vi "Main.vi"(11 "Module Admin":refnum<class "Delacor_lib_QMH_Module Admin.lvclass">) -> ()   [LabVIEW 2021, in "HMI.lvlib"]
doc: "This template is based off of the Queued Message Handler design pattern and the Queued Message Handler project template that ships with LabVIEW.\n\nThe main difference is that the queue is private to this module and communication between modules is performed via Broadcast and Request events.\n\nRequest events are wrapped in public API methods and are handled in the Event Handling Loop (EHL) of this VI. Any module can register for Broadcast events sent by this module. The EHL generates messages based on user interface actions.\n\nThe Message Handling Loop (MHL) processes messages generated by the EHL, or by other messages. The messages are string values, so new messages can be added easily to the Message Cases case structure in the MHL. Each message cluster can also provide an optional value for Message Data, which is a variant that can be converted to whatever message-specific data is required.\n_____\nBased on DQMH Dev Tools: Project Template 7.1.2.1547."
uses:
  HMI.lvlib
  <vilib>/Delacor/Delacor QMH/Libraries/Module Admin_class/Delacor_lib_QMH_Module Admin.lvclass
  Module Data--cluster.ctl
  Get Measurement from UDP HL--cluster.ctl
  Stop Argument--cluster.ctl
  <vilib>/Delacor/Delacor QMH/Libraries/Message Queue_class/Delacor_lib_QMH_Message Queue.lvclass/Delacor_lib_QMH_Message Queue.ctl
  <vilib>/Delacor/Delacor QMH/Libraries/Module Admin_class/Delacor_lib_QMH_Module Admin.lvclass/Delacor_lib_QMH_Module Admin.ctl
  Open UDP Connection Argument--cluster.ctl
  <vilib>/Utility/miscctls.llb/LVPointTypeDef.ctl
  <vilib>/Delacor/Delacor QMH/Libraries/Message Queue_class/Delacor_lib_QMH_Enqueue Message (Single).vi
  <vilib>/Delacor/Delacor QMH/Libraries/Module Admin_class/Delacor_lib_QMH_Get External Launch.vi
  <vilib>/Delacor/Delacor QMH/Libraries/Message Queue_class/Delacor_lib_QMH_Message Queue.lvclass
panel:
  out "CPU 2 (%)":u8(slide) scale=0.0..100.0
  out "CPU 1 (%)":u8(slide) scale=0.0..100.0
  out "Memory ROM Available (%)":u8(slide) scale=0.0..100.0
  out "Memory RAM Available (%)":u8(slide) scale=0.0..100.0
  out "Record Time":dbl format="%<%H:%M:%S%3u>t"
  in  "Record TDMS File":bool
  out "Analog Input":dbl[](array[numeric])
  out "Digital Input":bool[](array[boolean])
  out "error out":errorcluster
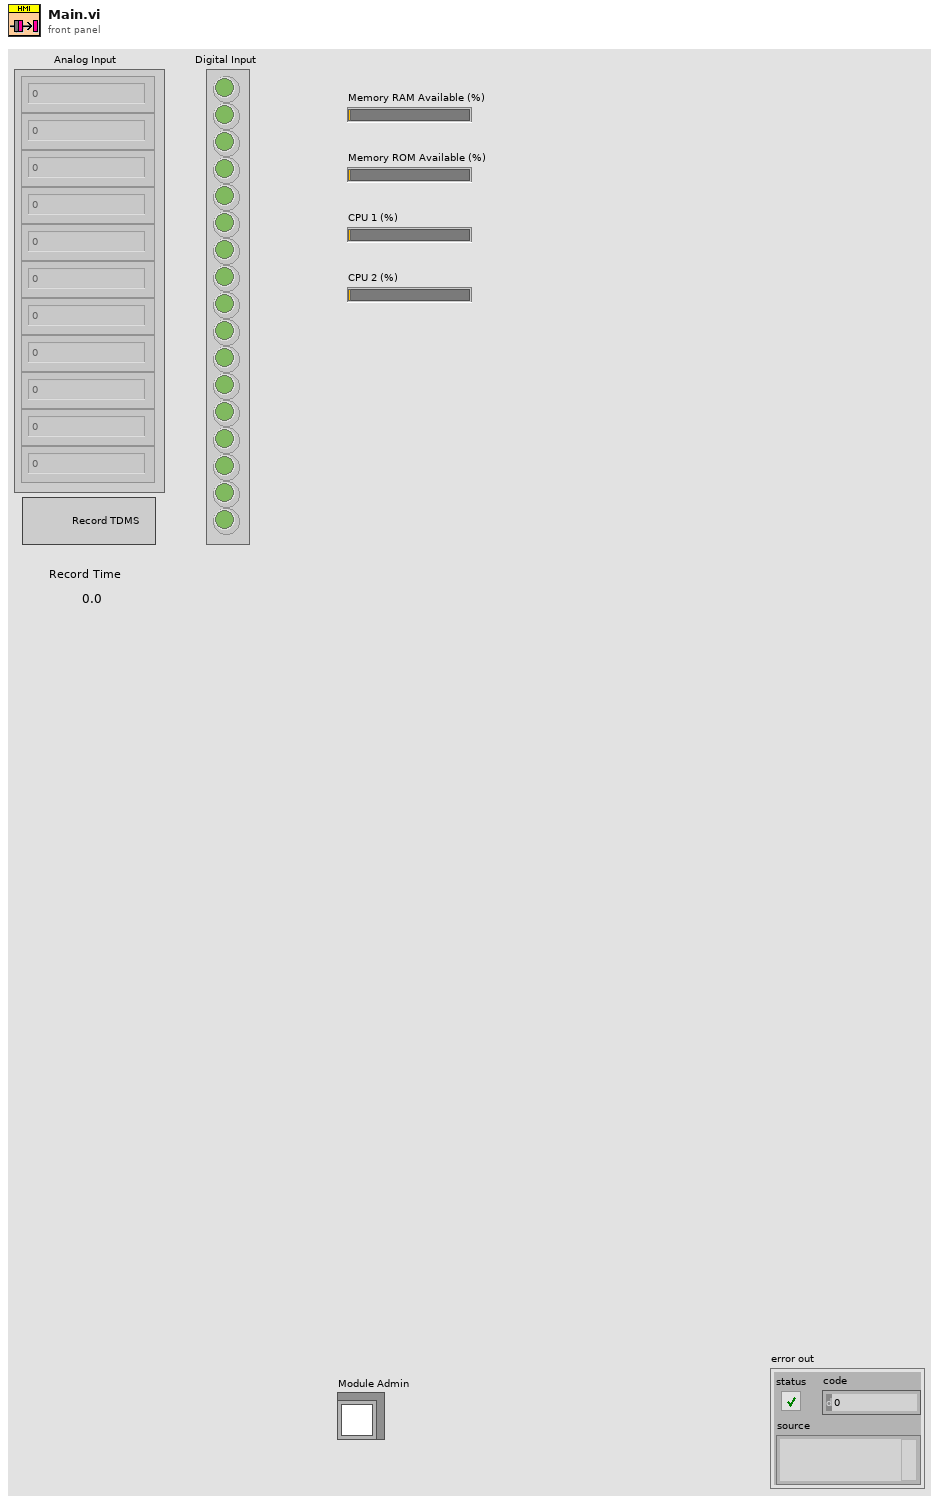
[diagram p1: front panel]
types:
  T1 = typedef "HMI.lvlib/Request Events--cluster.ctl" = cluster{"Stop Module":refnum<user-event>, "Show Panel":refnum<user-event>, "Hide Panel":refnum<user-event>, "Get Module Execution Status":refnum<user-event>, "Show Diagram":refnum<user-event>, "Private.Open UDP Connection":refnum<user-event>, "Private.Get UDP Info":refnum<user-event>, "Private.Recording":refnum<user-event>}
  T2 = typedef "HMI.lvlib/Get Measurement from UDP HL--cluster.ctl" = cluster{"IP RT":string, "Port RT":u16, "Port Host":u16, "connection ID":refnum<k16>, "Recording?":bool, "Timestamp":timestamp}
  T3 = typedef "HMI.lvlib/Module Data--cluster.ctl" = cluster{"Status":string, "IP RT":string, "Port RT":u16, "Port Host":u16, "connection ID":refnum<k16>}
  T4 = enum32{"invalid lock state", "Not Locked", "Locked (No Password)", "Password-protected"}
  T5 = typedef "HMI.lvlib/Stop Argument--cluster.ctl" = cluster{"Origin":string, "Exit via Stop Module Req?":bool, "Wait for Module to stop?":bool}
  T6 = typedef "HMI.lvlib/Open UDP Connection Argument--cluster.ctl" = cluster{"Boolean":bool}
  T7 = typedef "LVPointTypeDef.ctl" = cluster{"Horizontal":i16, "Vertical":i16}
  T8 = enum32{"Invalid", "Standard", "Closed", "Hidden", "Minimized", "Maximized"}
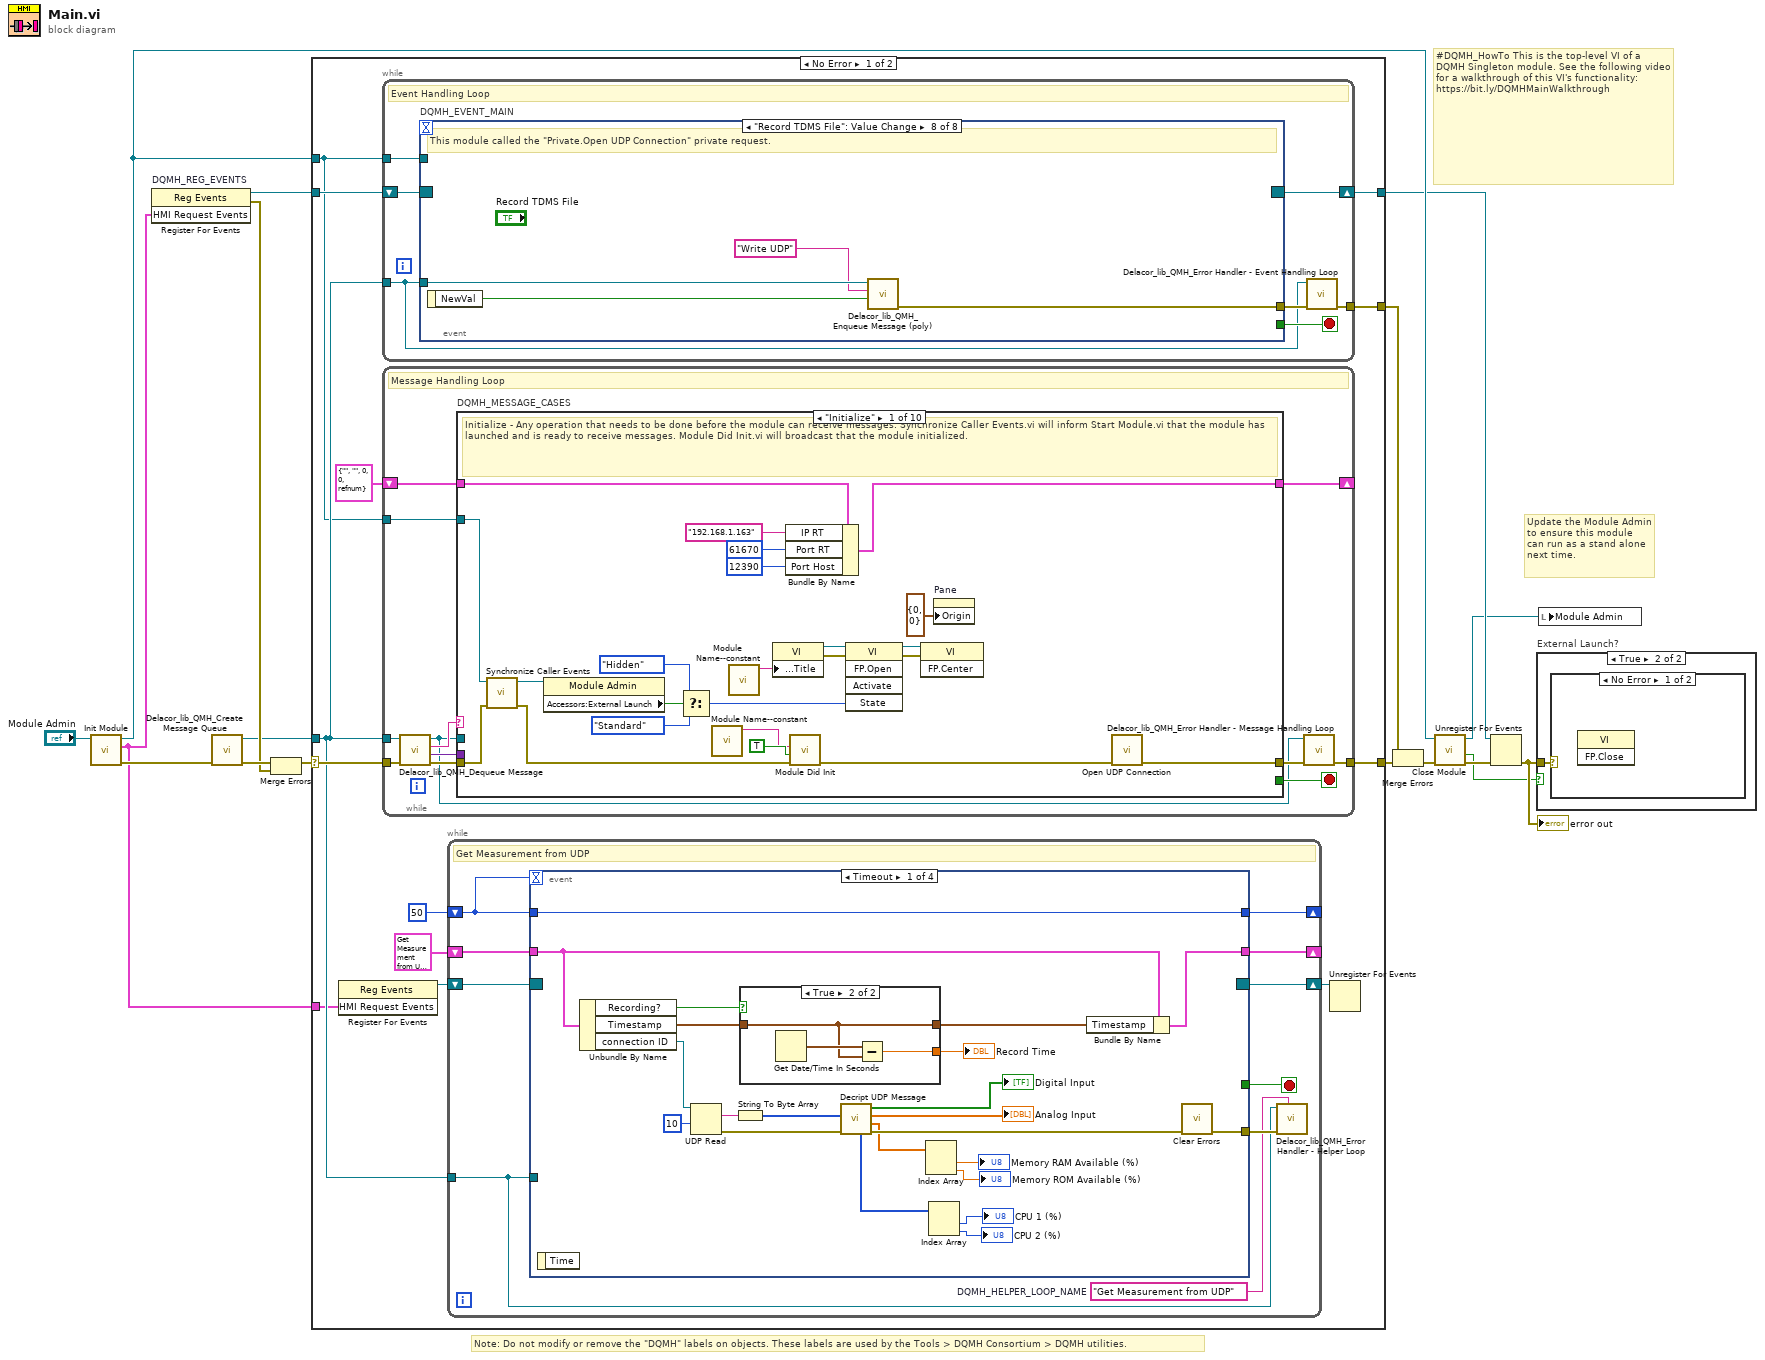
[diagram p0: block diagram]
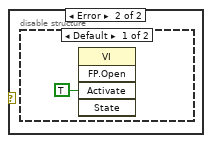
[diagram p3: hidden frame]
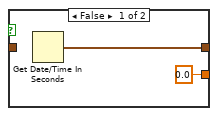
[diagram p5: hidden frame]
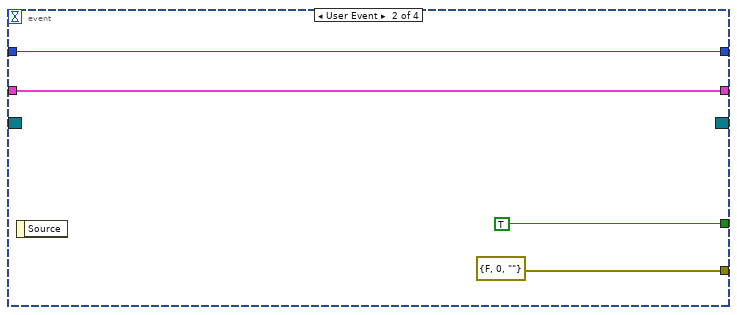
[diagram p6: hidden frame]
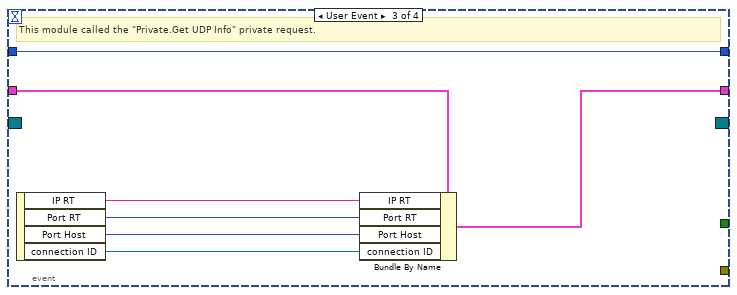
[diagram p7: hidden frame]
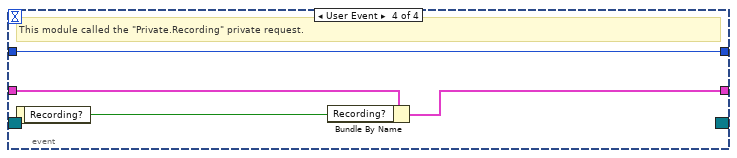
[diagram p8: hidden frame]
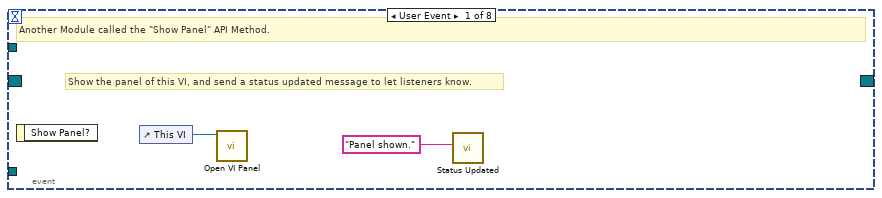
[diagram p9: hidden frame]
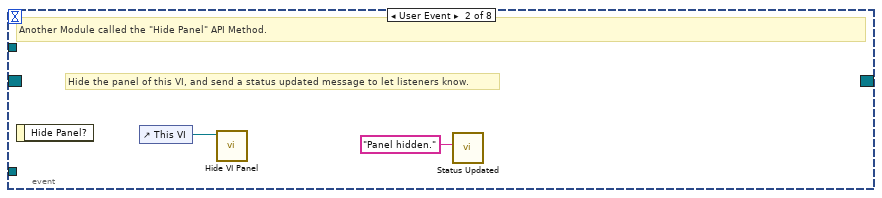
[diagram p10: hidden frame]
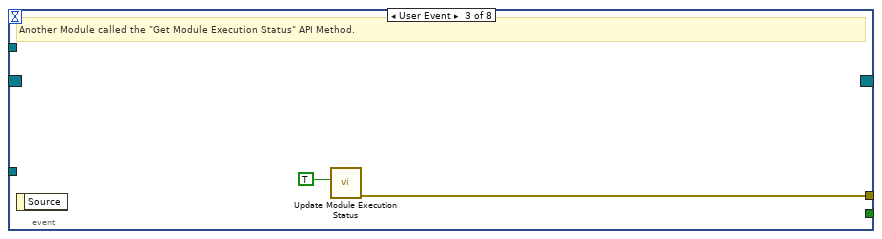
[diagram p11: hidden frame]
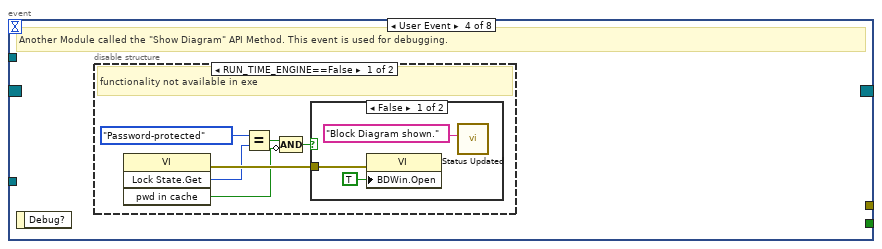
[diagram p12: hidden frame]
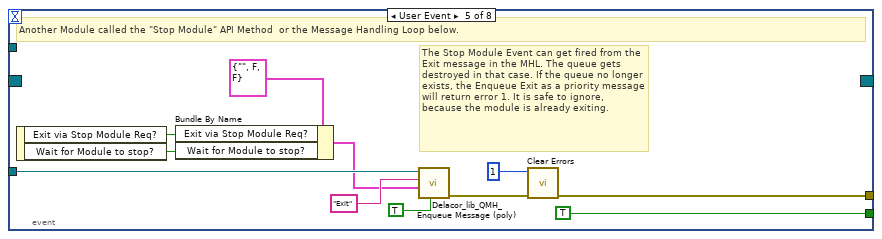
[diagram p15: hidden frame]
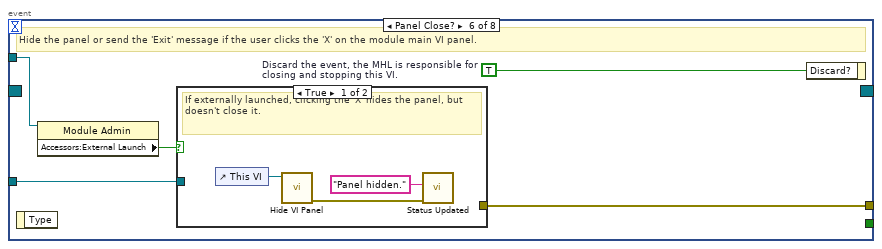
[diagram p16: hidden frame]
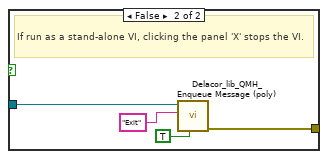
[diagram p17: hidden frame]
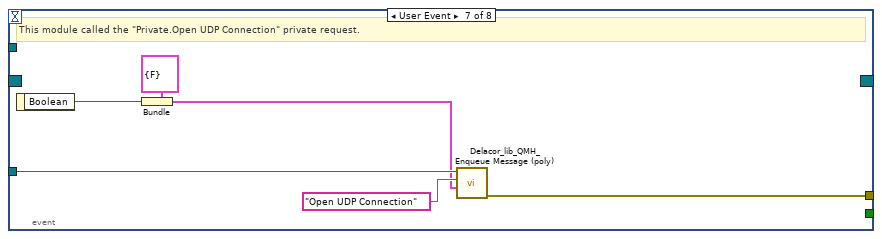
[diagram p18: hidden frame]
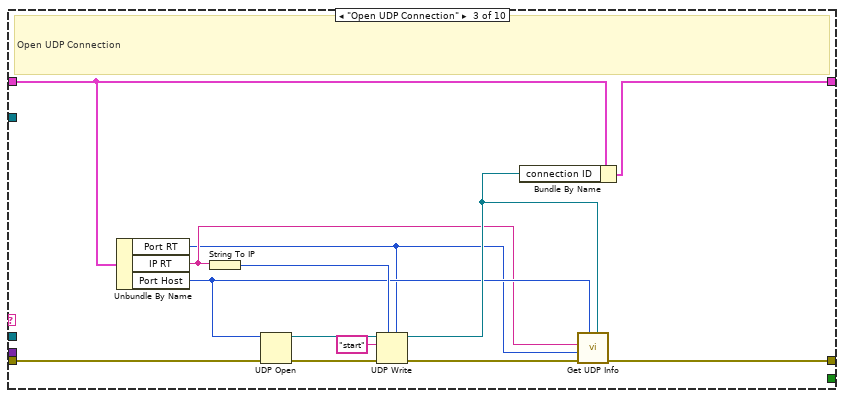
[diagram p20: hidden frame]
diagram:
  # "#DQMH_HowTo This is the top-level VI of a DQMH Singleton module. See the following video for a walkthrough of this VI's functionality: https://bit.ly/DQMHMainWalkthrough"
  # "Note: Do not modify or remove the \"DQMH\" labels on objects. These labels are used by the Tools > DQMH Consortium > DQMH utilities."
  # "Update the Module Admin to ensure this module can run as a stand alone next time."
  n1 = call "Init Module.vi"("Singleton Module Admin in"="Module Admin") -> ("error out"=w16:errorcluster, "HMI Request Events"=w1:T1, "Singleton Module Admin out"=w8:refnum<class "Delacor_lib_QMH_Module Admin.lvclass">)  [unwired: 8 in]
  n2 = register-events "DQMH_REG_EVENTS"(w1) -> (reference out=w6:refnum<event-registration>, error out=w9:errorcluster)  [unwired: 2 in]
  n3 = call <vilib>:"Delacor_lib_QMH_Create Message Queue.vi"("error in"=w16) -> ("error out"=w11:errorcluster, "Message Queue"=w5:refnum<class "Delacor_lib_QMH_Message Queue.lvclass">)  [unwired: 9 in]
  n4 = Merge Errors(w11, w9) -> (w10:errorcluster)
  n5 = case shown="No Error" w10 {
    selector: w10 -> [w28 w266]
    tunnel: [w30 w265] -> w17
    tunnel: [w27 w264] -> w7
    tunnel: w6 -> [w25 w264]
    tunnel: w5 -> [w24 w259]
    tunnel: [w29 _] -> w14
    tunnel: w8 -> [w23 w260]
    tunnel: w1 -> [w22 _]
    frame No Error {
      n6 = register-events ("DQMH_HELPER_REGFOREVENTS")(w22) -> (reference out=w20:refnum<event-registration>)  [unwired: 2 in, 1 out]
      n7 = while {
        tunnel: w24 -> [w83]
        shift-right: [w86] -> w27
        shift-left: w25 -> [w87]
        tunnel: [w88] -> w29
        tunnel: w23 -> [w84]
        stop <- w85 stop-if-true
        # "Event Handling Loop"
        n8 = event "DQMH_EVENT_MAIN" shown="[7] \"Record TDMS File\": Value Change" {
          selector: w87 -> [_ _ _ _ _ _ _ _]
          dyn-events: [_ _ _ _ _ _ _ _] -> w86
          timeout: _ -> [_ _ _ _ _ _ _ _]
          tunnel: [_ _ _ _ TRUE ("Discard?") _ _ _] -> w85
          tunnel: w83 -> [_ _ _ _ w111 w118 w133 w137]
          tunnel: [_ _ w95 _ w114 w120 w128 w135] -> w89
          tunnel: w84 -> [_ _ _ _ _ w117 _ _]
          event User Event {
            # "Show the panel of this VI, and send a status updated message to let listeners know."
            # "Another Module called the \"Show Panel\" API Method."
            n9 = event-data() -> ()  [unwired: 1 in, 1 out]
            n10 = control-ref of="This VI"() -> (w91:refnum<vi>)
            n11 = call "Open VI Panel.vi"("VI"=w91) -> ()  [unwired: 10 in, 1 out]
            n12 = call "Status Updated.vi"("Status"="Panel shown." ("format string")) -> ()  [unwired: 10 in, 1 out]
          }
          event User Event {
            # "Hide the panel of this VI, and send a status updated message to let listeners know."
            # "Another Module called the \"Hide Panel\" API Method."
            n13 = event-data() -> ()  [unwired: 1 in, 1 out]
            n14 = control-ref of="This VI"() -> (w93:refnum<vi>)
            n15 = call "Hide VI Panel.vi"("VI"=w93) -> ()  [unwired: 10 in, 1 out]
            n16 = call "Status Updated.vi"("Status"="Panel hidden." ("format string")) -> ()  [unwired: 10 in, 1 out]
          }
          event User Event {
            # "Another Module called the \"Get Module Execution Status\" API Method."
            n17 = event-data() -> ()  [unwired: 1 in, 1 out]
            n18 = call "Update Module Execution Status.vi"("Running?"=TRUE) -> ("error out"=w95:errorcluster)  [unwired: 10 in]
          }
          event User Event {
            # "Another Module called the \"Show Diagram\" API Method. This event is used for debugging."
            n19 = event-data() -> ()  [unwired: 1 in, 1 out]
            n20 = disable-structure shown="RUN_TIME_ENGINE==False" {
              frame condition #0 (active) {
                # "functionality not available in exe"
                n21 = invoke on="Invoke Node" class="VI" method="Lock State.Get"() -> (error out=w101:errorcluster, "Get Lock State"=w100:T4, "pwd in cache"=w97:bool)  [unwired: 4 in, 1 out]
                n22 = Equal?(x=T4."Password-protected", y=w100) -> (x = y?=w98:bool)
                n23 = Compound Arithmetic op=AND(w98, invert w97) -> (w96:bool)
                n24 = case shown="False" w96 {
                  tunnel: w101 -> [w104 _]
                  frame False {
                    n25 = property on="Property Node" class="VI"(error in=w104, "BDWin.Open"=TRUE ("Block Diagram Window:Open")) -> ()  [unwired: 1 in, 2 out]
                    n26 = call "Status Updated.vi"("Status"="Block Diagram shown." ("format string")) -> ()  [unwired: 10 in, 1 out]
                  }
                  frame True {
                    # "Password-protected VI, and the password is not in the cache. Do not show the diagram."
                  }
                }
              }
              frame condition #1 {
              }
            }
          }
          event User Event {
            # "The Stop Module Event can get fired from the Exit message in the MHL. The queue gets destroyed in that case. If the queue no longer exists, the Enqueue Exit as a priority message will return error 1. It is safe to ignore, because the module is already exiting."
            # "Another Module called the \"Stop Module\" API Method  or the Message Handling Loop below."
            n27 = event-data() -> ("Exit via Stop Module Req?"=w107:bool, "Wait for Module to stop?"=w106:bool)  [unwired: 1 in]
            n28 = Bundle By Name(cluster=T5 {"Origin"="", "Exit via Stop Module Req?"=FALSE, "Wait for Module to stop?"=FALSE} ("Stop Argument"), "Exit via Stop Module Req?"=w107, "Wait for Module to stop?"=w106) -> (w105:T5)
            n29 = call-poly <vilib>:"Delacor_lib_QMH_Enqueue Message (poly).vi"("Priority Message? (F)"=TRUE, "Message Data"=w105, "Message"="Exit", "Message Queue in"=w111) -> ("error out"=w115:errorcluster)  [unwired: 6 in, 1 out]
            n30 = call <vilib>:"Clear Errors.vi"("error in (no error)"=w115, "specific error code to clear (0: all)"=1) -> ("error out"=w114:errorcluster)  [unwired: 4 in, 1 out]
          }
          event Panel Close? {
            w119 = TRUE  # Discard the event, the MHL is responsible for closing and stopping this VI.
            # "Hide the panel or send the 'Exit' message if the user clicks the 'X' on the module main VI panel."
            n31 = event-data() -> ()  [unwired: 1 in, 1 out]
            n32 = property on="Property Node" class="Module Admin"(reference=w117) -> ("Accessors:External Launch"=w116:bool)  [unwired: 1 in, 2 out]
            n33 = case shown="True" w116 {
              tunnel: w118 -> [_ w126]
              tunnel: [_ w127] -> w120
              frame True {
                # "If externally launched, clicking the 'X' hides the panel, but doesn't close it."
                n34 = control-ref of="This VI"() -> (w123:refnum<vi>)
                n35 = call "Hide VI Panel.vi"("VI"=w123) -> ("error out"=w121:errorcluster)  [unwired: 10 in]
                n36 = call "Status Updated.vi"("error in"=w121, "Status"="Panel hidden." ("format string")) -> ()  [unwired: 9 in, 1 out]
              }
              frame False {
                # "If run as a stand-alone VI, clicking the panel 'X' stops the VI."
                n37 = call-poly <vilib>:"Delacor_lib_QMH_Enqueue Message (poly).vi"("Priority Message? (F)"=TRUE, "Message"="Exit", "Message Queue in"=w126) -> ("error out"=w127:errorcluster)  [unwired: 7 in, 1 out]
              }
            }
            n38 = event-data ("Event Filter Node")("Discard?"=w119) -> ()  [unwired: 1 in, 1 out]
          }
          event User Event {
            # "This module called the \"Private.Open UDP Connection\" private request."
            n39 = event-data() -> ("Boolean"=w129:bool)  [unwired: 1 in]
            n40 = Bundle(cluster=T6 {"Boolean"=FALSE} ("Open UDP Connection Argument"), "Boolean"=w129) -> (w130:T6)
            n41 = call-poly <vilib>:"Delacor_lib_QMH_Enqueue Message (poly).vi"("Message Data"=w130, "Message"="Open UDP Connection", "Message Queue in"=w133) -> ("error out"=w128:errorcluster)  [unwired: 7 in, 1 out]
          }
          event "Record TDMS File": Value Change {
            # "This module called the \"Private.Open UDP Connection\" private request."
            n42 = event-data() -> ("NewVal"=w134:bool)  [unwired: 1 in]
            n43 = call-poly <vilib>:"Delacor_lib_QMH_Enqueue Message (poly).vi"("Message Data"=w134, "Message"="Write UDP", "Message Queue in"=w137) -> ("error out"=w135:errorcluster)  [unwired: 7 in, 1 out]
          }
        }
        n44 = call-dynamic "Delacor_lib_QMH_Error Handler - Event Handling Loop.vi"("error in"=w89, "Message Queue in"=w83) -> ("dup error in"=w88:errorcluster)  [unwired: 8 in, 1 out]
      }
      n45 = while {
        tunnel: w24 -> [w138]
        shift-right: [w146] -> _
        shift-left: T3 {"Status"="", "IP RT"="", "Port RT"=0, "Port Host"=0, "connection ID"=refnum} ("Data Cluster") -> [w147]
        tunnel: w28 -> [w149]
        tunnel: [w141] -> w30
        tunnel: w23 -> [w142]
        stop <- w145 stop-if-true
        # "Message Handling Loop"
        n46 = call-dynamic "Delacor_lib_QMH_Dequeue Message.vi"("error in"=w149, "Message Queue in"=w138) -> ("error out"=w148:errorcluster, "Message Data"=w143:variant, "Message"=w144:string, "Message Queue out"=w139:refnum<class "Delacor_lib_QMH_Message Queue.lvclass">)  [unwired: 6 in]
        n47 = case "DQMH_MESSAGE_CASES" shown="\"Initialize\"" w144 {
          selector: w144 -> [_ _ _ _ _ _ _ _ _ w254]
          tunnel: w139 -> [_ _ _ _ _ _ _ w220 w242 _]
          tunnel: w148 -> [w170 w174 w187 w202 w205 w207 w216 w227 w248 w257]
          tunnel: [w155 w174 w179 w189 w204 w207 w215 w223 w243 w258] -> w140
          tunnel: w147 -> [w153 w173 w184 w201 w203 w206 w213 w222 w241 w255]
          tunnel: [w154 w173 w185 w201 w203 w206 w213 w222 w241 w255] -> w146
          tunnel: [_ _ _ _ _ _ _ _ w240 _] -> w145
          tunnel: w143 -> [_ _ _ w197 _ _ _ w221 w239 _]
          tunnel: w142 -> [w161 _ _ _ _ _ _ w219 w234 _]
          frame "Initialize" {
            # "Initialize - Any operation that needs to be done before the module can receive messages. Synchronize Caller Events.vi will inform Start Module.vi that the module has launched and is ready to receive messages. Module Did Init.vi will broadcast that the module initialized."
            n48 = call "Synchronize Caller Events.vi"("error in"=w170, "Singleton Module Admin in"=w161) -> ("error out"=w169:errorcluster, "Singleton Module Admin out"=w158:refnum<class "Delacor_lib_QMH_Module Admin.lvclass">)  [unwired: 8 in]
            n49 = property on="Property Node" class="Module Admin"(reference=w158) -> ("Accessors:External Launch"=w165:bool)  [unwired: 1 in, 2 out]
            n50 = Select(t=T8."Hidden" ("State"), s=w165, f=T8."Standard" ("State")) -> (s? t:f=w162:T8)
            n51 = call "Module Name--constant.vi"() -> ("Module Name"=w159:string)  [unwired: 11 in]
            n52 = call "Module Name--constant.vi"() -> ("Module Name"=w168:string)  [unwired: 11 in]
            n53 = property on="Property Node" class="VI"("Front Panel.Title"=w168) -> (reference out=w167:refnum<vi>, error out=w172:errorcluster)  [unwired: 2 in]
            n54 = Bundle By Name(cluster=w153, "IP RT"="192.168.1.163", "Port RT"=u16 61670, "Port Host"=u16 12390) -> (w154:T3)
            n55 = call "Module Did Init.vi"("error in"=w169, "Initialized?"=TRUE, "Origin"=w159) -> ("error out"=w156:errorcluster)  [unwired: 8 in]
            n56 = invoke on="Invoke Node" class="VI" method="FP.Open"(reference=w167, error in=w172, "State"=w162) -> (reference out=w166:refnum<vi>, error out=w171:errorcluster)  [unwired: 2 in, 3 out]
            n57 = invoke on="Invoke Node" class="VI" method="FP.Center"(reference=w166, error in=w171) -> ()  [unwired: 1 in, 3 out]
            n58 = property on="Pane" class="Pane"("Origin"=T7 {"Horizontal"=0, "Vertical"=0}) -> ()  [unwired: 2 in, 2 out]
            n59 = call "Open UDP Connection.vi"("error in"=w156) -> ("error out"=w155:errorcluster)  [unwired: 10 in]
          }
          frame "---Module Specific---" {
            # "Separator -- The following cases handle messages specific to this Module."
          }
          frame "Open UDP Connection" {
            # "Open UDP Connection"
            n60 = Unbundle By Name(w184) -> ("Port RT"=w175:u16, "IP RT"=w176:string, "Port Host"=w177:u16)
            n61 = String To IP(1:w176) -> (0:w181:u32)
            n62 = UDP Open(8:w187, 11:w177) -> (port=w183:refnum<k16>, 0:w186:errorcluster)  [unwired: 3 in, 1 out]
            n63 = UDP Write(address=w181, port or service name=w175, connection ID=w183, data in="start", 8:w186) -> (error out=w180:errorcluster, 3:w178:refnum<k16>)  [unwired: 1 in]
            n64 = Bundle By Name(cluster=w184, "connection ID"=w178) -> (w185:T3)
            n65 = call "Get UDP Info.vi"("connection ID"=w178, "Port Host"=w177, "error in"=w180, "Port RT"=w175, "IP RT"=w176) -> ("error out"=w179:errorcluster)  [unwired: 6 in]
          }
          frame "Write UDP" {
            # "Write UDP"
            n66 = Variant To Data(error in=w202, type=FALSE, Variant=w197) -> (data=w188:bool, error out=w199:errorcluster)
            n67 = Type Cast(type=u8[] [], x=w188) -> (*(type *) &x=w195:u8[])
            n68 = Byte Array To String(unsigned byte array=w195) -> (string=w194:string)
            n69 = Unbundle By Name(w201) -> ("Port RT"=w193:u16, "IP RT"=w192:string, "connection ID"=w200:refnum<k16>)
            n70 = String To IP(1:w192) -> (0:w191:u32)
            n71 = UDP Write(address=w191, port or service name=w193, connection ID=w200, data in=w194, 8:w199) -> (error out=w190:errorcluster)  [unwired: 1 in, 1 out]
            n72 = call "Recording.vi"("error in"=w190, "Recording?"=w188) -> ("error out"=w189:errorcluster)  [unwired: 9 in]
          }
          frame "---Copy This Frame---" {
            # "Duplicate this frame when creating new messages.  Change this comment in the duplicated frame to describe this message."
            n73 = Merge Errors(w205) -> (w204:errorcluster)
          }
          frame "---Exit and Error Handling---" {
            # "Separator - The following cases handle errors and exit messages."
          }
          frame "Simulate MHL Error" {
            # "#DQMH_HowTo The 'Simulate MHL Error' button  illustrates how the MHL handles errors. This event is instructional in nature and can be removed."
            # "Simulate an error occurring at the MHL"
            n74 = call "Module Name--constant.vi"() -> ("Module Name"=w209:string)  [unwired: 11 in]
            n75 = Format Into String(format string="Simulated error originating at Message Handling Loop in %s", w209) -> (resulting string=w210:string)  [unwired: 2 in, 1 out]
            n76 = call <vilib>:"Error Cluster From Error Code.vi"("show call chain? (False)"=TRUE, "error message (\"\")"=w210, "error code (0)"=5001) -> ("error out"=w214:errorcluster)  [unwired: 6 in]
            n77 = Merge Errors(w216, w214) -> (w215:errorcluster)
          }
          frame "Error" {
            # "#DQMH_CodeRecommended - If the module is running in standalone mode (External Launch = FALSE), this code will pop up an error dialog and call the 'Exit' message if an error occurs. Add more fine-grained error management here."
            # "Error - Check the error message data and respond accordingly. This message is sent by the \"Error Handler\" VIs at the end of each loop in this application."
            n78 = property on="Property Node" class="Module Admin"(reference=w219) -> ("Accessors:External Launch"=w218:bool)  [unwired: 1 in, 2 out]
            n79 = Variant To Data(error in=w227, type=errorcluster {"status"=FALSE, "code"=0, "source"=""} ("error constant"), Variant=w221) -> (data=w217:errorcluster, error out=w225:errorcluster)
            n80 = local write "error out"(w217) -> ()
            n81 = call "Error Reported.vi"("Error"=w217) -> ()  [unwired: 10 in, 1 out]
            n82 = case shown="False" w218 {
              tunnel: [w232 _] -> w224
              tunnel: w220 -> [w230 _]
              tunnel: w217 -> [w231 _]
              frame False {
                n83 = disable-structure shown="Default" {
                  disable-tunnel: w231 -> [w233 _]
                  frame condition #0 (active) {
                    # "If the module is running standalone, then pop up an error dialog and call the \"Exit\" message."
                    n84 = call <vilib>:"Simple Error Handler.vi"("error in (no error)"=w233) -> ()  [unwired: 4 in, 5 out]
                  }
                  frame condition #1 {
                    # "To prevent the Simple Error Handler VI from being loaded (e.g. when deploying to a Real-Time target), add the Conditional Disable Symbol \"DQMH_Disable_SEH\" to your project and set it to TRUE."
                  }
                }
                n85 = call-poly <vilib>:"Delacor_lib_QMH_Enqueue Message (poly).vi"("Priority Message? (F)"=TRUE, "Message"="Exit", "Message Queue in"=w230) -> ("error out"=w232:errorcluster)  [unwired: 7 in, 1 out]
              }
              frame True {
                # "If the module was launched externally, calling the Error Reported broadcast VI is the only action performed by the \"Error\" message. The module's caller can then process the error appropriately."
              }
            }
            n86 = Merge Errors(w225, w224) -> (w223:errorcluster)
          }
          frame "Exit" {
            w238 = 91  # 91: not all Exit messages will have an argument
            w240 = TRUE  # Stop the VI
            # "Release the message queue reference"
            # "#DQMH_CodeNeeded - Add any required cleanup code here."
            # "Exit - Exit the application."
            n87 = Variant To Data(error in=w248, type=T5 {"Origin"="", "Exit via Stop Module Req?"=FALSE, "Wait for Module to stop?"=FALSE} ("Stop Argument"), Variant=w239) -> (data=w236:T5, error out=w245:errorcluster)
            n88 = call <vilib>:"Clear Errors.vi"("error in (no error)"=w245, "specific error code to clear (0: all)"=w238) -> ("error out"=w247:errorcluster)  [unwired: 4 in, 1 out]
            n89 = control-ref of="This VI"() -> (w235:refnum<vi>)
            n90 = call-dynamic "Delacor_lib_QMH_Release Message Queue.vi"("error in"=w247, "Message Queue"=w242) -> ("error out"=w246:errorcluster)  [unwired: 9 in]
            n91 = call "Handle Exit.vi"("Stop Argument"=w236, "Admin in"=w234, "VI reference"=w235) -> ("error out"=w244:errorcluster)  [unwired: 7 in, 1 out]
            n92 = Merge Errors(w246, w244) -> (w243:errorcluster)
            n93 = call "Error Reported.vi"("Error"=w243) -> ()  [unwired: 10 in, 1 out]
          }
          frame Default {
            # "'Default' case only runs if there is a message that isn't defined in any of the other cases.  Output a programming error."
            n94 = call "Module Name--constant.vi"() -> ("Module Name"=w253:string)  [unwired: 11 in]
            n95 = Format Into String(format string="The invalid message string \"%s\" was received in the Message Handling Loop for module \"%s\".", w254, w253) -> (resulting string=w249:string)  [unwired: 2 in, 1 out]
            n96 = call <vilib>:"Error Cluster From Error Code.vi"("show call chain? (False)"=TRUE, "error message (\"\")"=w249, "error code (0)"=1) -> ("error out"=w256:errorcluster)  [unwired: 6 in]
            n97 = Merge Errors(w257, w256) -> (w258:errorcluster)
          }
        }
        n98 = call-dynamic "Delacor_lib_QMH_Error Handler - Message Handling Loop.vi"("error in"=w140, "Message Queue in"=w139) -> ("dup error in"=w141:errorcluster)  [unwired: 8 in, 1 out]
      }
      n99 = while "DQMH_HELPER_LOOP" {
        shift-right: [w40] -> _
        shift-left: 50 -> [w39]
        shift-right: [w37] -> w21
        shift-left: w20 -> [w38]
        tunnel: w24 -> [w34]
        shift-right: [w32] -> _
        shift-left: T2 {"IP RT"="", "Port RT"=0, "Port Host"=0, "connection ID"=refnum, "Recording?"=FALSE, "Timestamp"=timestamp(0 s since 1904-01-01)} ("Get Measurement from UDP HL--cluster") -> [w31]
        stop <- w36 stop-if-true
        w33 = "Get Measurement from UDP"  # DQMH_HELPER_LOOP_NAME
        # "Get Measurement from UDP"
        n100 = event "DQMH_HELPER_EVENT_STRUCTURE" shown="[0] Timeout" {
          selector: w38 -> [_ _ _ _]
          dyn-events: [_ _ _ _] -> w37
          timeout: w39 -> [_ _ _ _]
          tunnel: w39 -> [w62 w71 w78 w82]
          tunnel: [w62 w71 w78 w82] -> w40
          tunnel: [_ TRUE _ _] -> w36
          tunnel: [w59 errorcluster {"status"=FALSE, "code"=0, "source"=""} ("error constant") _ _] -> w35
          tunnel: w34 -> [_ _ _ _]
          tunnel: [w42 w68 w72 w80] -> w32
          tunnel: w31 -> [w46 w68 w77 w81]
          event Timeout {
            n101 = event-data() -> ()  [unwired: 1 in, 1 out]
            n102 = Unbundle By Name(w46) -> ("Recording?"=w45:bool, "Timestamp"=w44:timestamp, "connection ID"=w43:refnum<k16>)
            n103 = UDP Read(connection ID=w43, timeout ms (25000)=10) -> (data out=w60:string, error out=w57:errorcluster)  [unwired: 2 in, 3 out]
            n104 = String To Byte Array(string=w60) -> (unsigned byte array=w58:u8[])
            n105 = case shown="True" w45 {
              tunnel: [w64 w66] -> w41
              tunnel: w44 -> [_ w66]
              tunnel: [0.0 w65] -> w53
              frame False {
                n106 = Get Date/Time In Seconds() -> (seconds since 1Jan1904=w64:timestamp)
              }
              frame True {
                n107 = Get Date/Time In Seconds() -> (seconds since 1Jan1904=w67:timestamp)
                n108 = Subtract(x=w67, y=w66) -> (x-y=w65:dbl)
              }
            }
            "Record Time" <- w53
            n109 = call "Decript UDP Message.vi"("Error In"=w57, "UDP Message"=w58) -> ("Error Out"=w56:errorcluster, "Memory"=w52:dbl[], "Analog Input"=→"Analog Input":dbl[], "Digital Input"=→"Digital Input":bool[], "CPU"=w49:u32[])  [unwired: 5 in]
            n110 = Index Array(array=w52) -> (element #1=→"Memory RAM Available (%)":dbl, element #2=→"Memory ROM Available (%)":dbl)  [unwired: 2 in]
            n111 = Index Array(array=w49) -> (element #1=→"CPU 1 (%)":u32, element #2=→"CPU 2 (%)":u32)  [unwired: 2 in]
            n112 = Bundle By Name(cluster=w46, "Timestamp"=w41) -> (w42:T2)
            n113 = call <vilib>:"Clear Errors.vi"("error in (no error)"=w56) -> ("error out"=w59:errorcluster)  [unwired: 5 in, 1 out]
          }
          event User Event {
            n114 = event-data() -> ()  [unwired: 1 in, 1 out]
          }
          event User Event {
            # "This module called the \"Private.Get UDP Info\" private request."
            n115 = event-data() -> ("IP RT"=w76:string, "Port RT"=w75:u16, "Port Host"=w74:u16, "connection ID"=w73:refnum<k16>)  [unwired: 1 in]
            n116 = Bundle By Name(cluster=w77, "IP RT"=w76, "Port RT"=w75, "Port Host"=w74, "connection ID"=w73) -> (w72:T2)
          }
          event User Event {
            # "This module called the \"Private.Recording\" private request."
            n117 = event-data() -> ("Recording?"=w79:bool)  [unwired: 1 in]
            n118 = Bundle By Name(cluster=w81, "Recording?"=w79) -> (w80:T2)
          }
        }
        n119 = call-dynamic "Delacor_lib_QMH_Error Handler - Helper Loop.vi"("Error Debug"=w33, "error in"=w35, "Message Queue in"=w34) -> ()  [unwired: 7 in, 2 out]
      }
      n120 = Unregister For Events(event registration refnum=w21) -> ()  [unwired: 1 in, 1 out]
    }
    frame Error {
      # "Synchronize Caller Events.vi will inform Start Module.vi that the module has launched and will let the code calling Start Module.vi register for broadcasts and would permit the caller receive the broadcast that an error occurred at launch time."
      n121 = call-dynamic "Delacor_lib_QMH_Release Message Queue.vi"("error in"=w266, "Message Queue"=w259) -> ("error out"=w265:errorcluster)  [unwired: 9 in]
      n122 = call "Synchronize Caller Events.vi"("Singleton Module Admin in"=w260) -> ("error out"=w267:errorcluster)  [unwired: 9 in, 1 out]
      n123 = call "Module Name--constant.vi"() -> ("Module Name"=w263:string)  [unwired: 11 in]
      n124 = Format Into String(format string="An error occurred during initialization. %s is no longer running.", w263) -> (resulting string=w261:string)  [unwired: 2 in, 1 out]
      n125 = Merge Errors(w265, w267) -> (w268:errorcluster)
      n126 = call "Error Reported.vi"("Additional Information"=w261, "Error"=w268) -> ()  [unwired: 9 in, 1 out]
    }
  }
  n127 = Merge Errors(w14, w17) -> (w13:errorcluster)
  n128 = call "Close Module.vi"("error in"=w13, "Module Admin in"=w8) -> ("error out"=w15:errorcluster, "External Launch"=w2:bool, "Module Admin out"=w3:refnum<class "Delacor_lib_QMH_Module Admin.lvclass">)  [unwired: 7 in]
  n129 = Unregister For Events(event registration refnum=w7, error in=w15) -> (error out=w12:errorcluster)
  "error out" <- w12
  n130 = case "External Launch?" shown="True" w2 {
    tunnel: w12 -> [_ w269]
    frame False {
    }
    frame True {
      n131 = case shown="No Error" w269 {
        frame No Error {
          n132 = invoke on="Invoke Node" class="VI" method="FP.Close"() -> ()  [unwired: 3 in, 3 out]
        }
        frame Error {
          n133 = disable-structure shown="Default" {
            frame condition #0 (active) {
              n134 = invoke class="VI" method="FP.Open"("Activate"=TRUE ("Activate?")) -> ()  [unwired: 4 in, 5 out]
            }
            frame condition #1 {
              # "Don't show panel on error if running inside a built EXE."
            }
          }
        }
      }
    }
  }
  n135 = local write "Module Admin"(w3) -> ()
